vi "TTi MX100 Output DC Volts.vi"() -> ()   [LabVIEW 2025]
doc: "This example shows how to configure the instrument's output voltage level, over current protection, and over voltage protection. The actual voltage level and actual current level are returned as well as whether over voltage protection (OVP) or over current protection (OCP) has been tripped."
uses:
  <instrlib>/TTi-MX100/TTi MX100.lvlib
panel:
  in  "Serial Configuration":T1={"Baud Rate"=9600, "Parity"=0, "Data Bits"=8, "Stop Bits"=10, "Flow Control"=0} {"Flow Control" items=["None", "XON/XOFF", "RTS/CTS", "XON/XOFF & RTS/CTS", "DTR/DSR", "XON/XOFF & DTR/DSR"]; "Stop Bits" items=["1.0"=10, "1.5"=15, "2.0"=20]; "Data Bits" items=["7"=7, "8"=8]; "Parity" items=["None", "Odd", "Even", "Mark", "Space"]; "Baud Rate" items=["300"=300, "600"=600, "1200"=1200, "2400"=2400, "4800"=4800, "9600"=9600, "19200"=19200]}
  in  "Stop Output":bool
  out "OCP Tripped":bool
  out "OVP Tripped":bool
  in  "Voltage Limit (0V)":dbl format="%.2f"
  out "Output Current  (A)":dbl format="%.2f"
  out "Output Voltage  (V)":dbl format="%.2f"
  in  "Voltage Level (0.0 V)":dbl format="%.2f"
  in  "Current Limit (0A)":dbl format="%.2f"
  in  "Channel (1:Channel 1)":i32(ring)=1 items=["Channel 1"=1, "Channel 2"=2]
  in  "VISA resource name":refnum<visa-resource-name>
  # "(c) 2014 <Enter Company Name Here>.  ALL RIGHTS RESERVED."
  # "Over Voltage Protection"
  # "Over Current Protection"
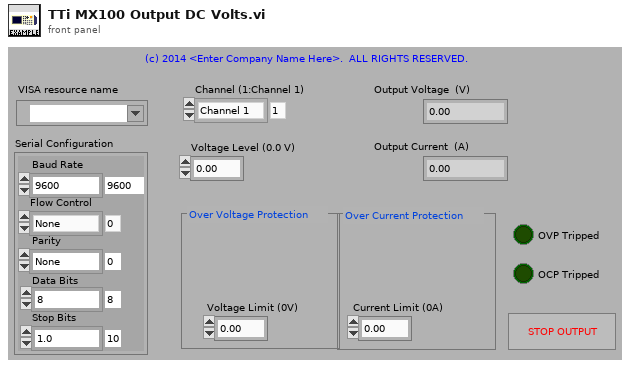
[diagram p1: front panel]
types:
  T1 = cluster{"Baud Rate":u32, "Parity":u16, "Data Bits":u16, "Stop Bits":u16, "Flow Control":u16}
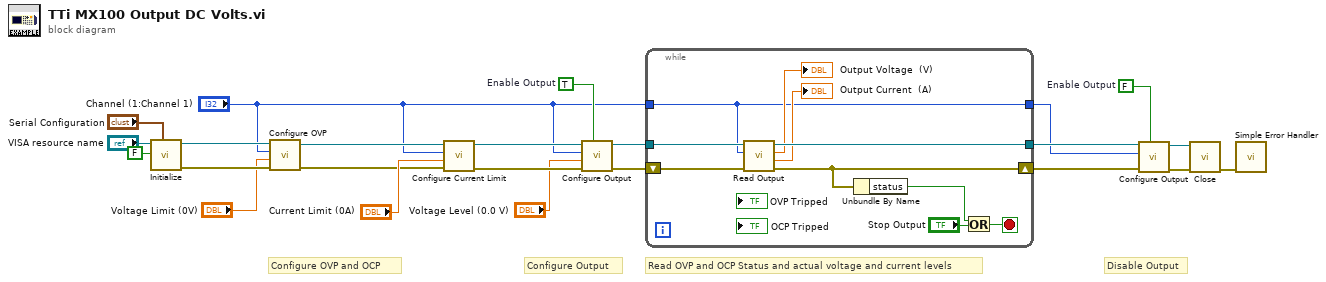
[diagram p0: block diagram]
diagram:
  w11 = FALSE  # Enable Output
  w12 = TRUE  # Enable Output
  # "Disable Output"
  # "Read OVP and OCP Status and actual voltage and current levels"
  # "Configure Output"
  # "Configure OVP and OCP"
  n1 = call <instrlib>:"Initialize.vi"("Serial Configuration"="Serial Configuration", "ID Query (True)"=FALSE, "VISA resource name"="VISA resource name") -> ("error out"=w8:errorcluster, "VISA resource name out"=w9:refnum<visa-resource-name>)  [unwired: 7 in]
  n2 = call <instrlib>:"Configure OVP.vi"("error in (no error)"=w8, "Voltage Limit (0.0 V)"="Voltage Limit (0V)", "Channel (1: Channel 1)"="Channel (1:Channel 1)", "VISA resource name"=w9) -> ("error out"=w7:errorcluster, "VISA resource name out"=w6:refnum<visa-resource-name>)  [unwired: 6 in]
  n3 = call <instrlib>:"Configure Current Limit.vi"("error in (no error)"=w7, "Current Limit (0.0 A)"="Current Limit (0A)", "Channel (1: Channel 1)"="Channel (1:Channel 1)", "VISA resource name"=w6) -> ("error out"=w21:errorcluster, "VISA resource name out"=w22:refnum<visa-resource-name>)  [unwired: 6 in]
  n4 = call <instrlib>:"Configure Output.vi"("Enable Output (T: Enable)"=w12, "error in (no error)"=w21, "Voltage Level (0.0 V)"="Voltage Level (0.0 V)", "Channel (1: Channel 1)"="Channel (1:Channel 1)", "VISA resource name"=w22) -> ("error out"=w18:errorcluster, "VISA resource name out"=w19:refnum<visa-resource-name>)  [unwired: 5 in]
  n5 = while {
    tunnel: w19 -> [w32]
    tunnel: [w33] -> w17
    tunnel: "Channel (1:Channel 1)" -> [w28]
    tunnel: [w28] -> w3
    shift-right: [w25] -> w16
    shift-left: w18 -> [w31]
    stop <- w27 stop-if-true
    n6 = call <instrlib>:"Read Output.vi"("error in (no error)"=w31, "Channel (1: Channel 1)"=w28, "VISA resource name"=w32) -> ("error out"=w25:errorcluster, "Actual Current Level (A)"=→"Output Current  (A)":dbl, "Actual Voltage Level (V)"=→"Output Voltage  (V)":dbl, "VISA resource name out"=w33:refnum<visa-resource-name>)  [unwired: 5 in]
    n7 = Unbundle By Name(w25) -> ("status"=w24:bool)
    n8 = Or(x=w24, y="Stop Output") -> (x .or. y?=w27:bool)
  }
  n9 = call <instrlib>:"Configure Output.vi"("Enable Output (T: Enable)"=w11, "error in (no error)"=w16, "Channel (1: Channel 1)"=w3, "VISA resource name"=w17) -> ("error out"=w14:errorcluster, "VISA resource name out"=w15:refnum<visa-resource-name>)  [unwired: 6 in]
  n10 = call <instrlib>:"Close.vi"("error in (no error)"=w14, "VISA resource name"=w15) -> ("error out"=w10:errorcluster)  [unwired: 9 in]
  n11 = call <vilib>:"Simple Error Handler.vi"("error in (no error)"=w10) -> ()  [unwired: 4 in, 5 out]
